vi "test lvjson round trip.vi"(8 "error in (no error)":errorcluster) -> (0 "error out":errorcluster)   [LabVIEW 2019, in "labview_json_tests.lvlib"]
uses:
  labview_json_tests.lvlib
  lib/labview_json.lvlib
panel:
  out "String":string
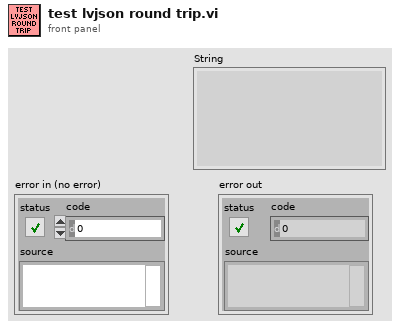
[diagram p1: front panel]
types:
  T1 = typedef "labview_json.lvlib/Element.ctl" = cluster{"Key":string, "Type":T2, "Value":variant}
  T2 = typedef "labview_json.lvlib/Element Type.ctl" = enum8{"NULL", "OBJECT", "ARRAY", "BOOL", "INT", "UINT", "FLOAT", "STRING"}
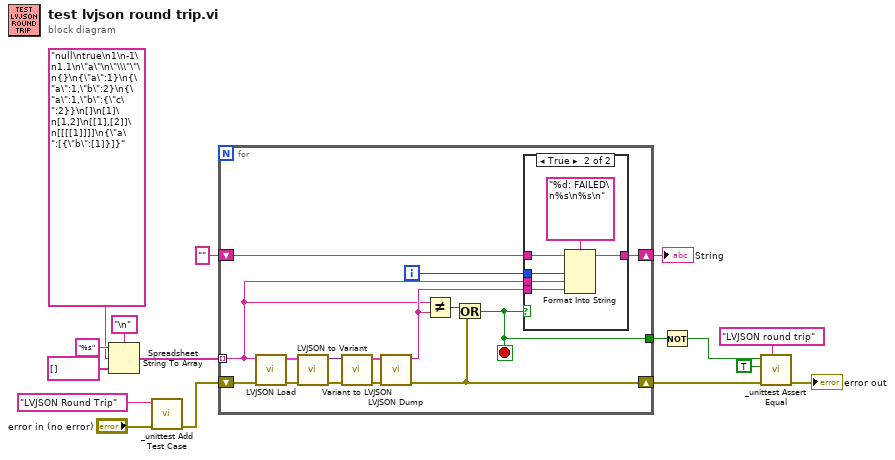
[diagram p0: block diagram]
diagram:
  n1 = Spreadsheet String To Array(delimiter (Tab)="\n", format string="%s", spreadsheet string="null\ntrue\n1\n-1\n1.1\n\"a\"\n\"\\\"\"\n{}\n{\"a\":1}\n{\"a\":1,\"b\":2}\n{\"a\":1,\"b\":{\"c\":2}}\n[]\n[1]\n[1,2]\n[[1],[2]]\n[[[[1]]]]\n{\"a\":[{\"b\":[1]}]}" ("JSON in"), array type (2D Dbl)=string[] []) -> (array=w8:string[])
  n2 = call "_unittest Add Test Case.vi"("error in (no error)"="error in (no error)", "Test Case"="LVJSON Round Trip") -> ("error out"=w6:errorcluster)  [unwired: 9 in]
  n3 = for {
    tunnel: w8 -> [w18] mode=indexing
    shift-right: [w23] -> w1
    shift-left: "" -> [w22]
    shift-right: [w20] -> w5
    shift-left: w6 -> [w19]
    tunnel: [w17] -> w3
    i -> [w24]
    stop <- w17 stop-if-true
    n4 = call "LVJSON Load.vi"("error in (no error)"=w19, "JSON in"=w18) -> ("error out"=w30:errorcluster, "Root Element out"=w31:T1)  [unwired: 8 in]
    n5 = call "LVJSON to Variant.vi"("error in (no error)"=w30, "Root Element in"=w31) -> ("error out"=w28:errorcluster, "Variant out"=w29:variant)  [unwired: 7 in, 1 out]
    n6 = call "Variant to LVJSON.vi"("error in (no error)"=w28, "Variant in"=w29) -> ("error out"=w26:errorcluster, "Element out"=w27:T1)  [unwired: 8 in]
    n7 = call "LVJSON Dump.vi"("error in (no error)"=w26, "Root Element in"=w27) -> ("error out"=w20:errorcluster, "JSON out"=w25:string)  [unwired: 7 in, 1 out]
    n8 = Not Equal?(x=w18, y=w25) -> (x != y?=w21:bool)
    n9 = Or(x=w21, y=w20) -> (x .or. y?=w17:bool)
    n10 = case shown="True" w17 {
      tunnel: w18 -> [_ w38]
      tunnel: w25 -> [_ w37]
      tunnel: w24 -> [_ w35]
      tunnel: [w32 w34] -> w23
      tunnel: w22 -> [w32 w33]
      frame False {
      }
      frame True {
        n11 = Format Into String(format string="%d: FAILED\n%s\n%s\n", initial string=w33, w35, w38, w37) -> (resulting string=w34:string)  [unwired: 1 in, 1 out]
      }
    }
  }
  "String" <- w1
  n12 = Not(x=w3) -> (.not. x?=w2:bool)
  n13 = call "_unittest Assert Equal.vi"("Message"="LVJSON round trip", "error in (no error)"=w5, "Expected Value"=TRUE, "Actual Value"=w2) -> ("error out"=→"error out":errorcluster)  [unwired: 7 in]
